vi "Go_To_Level.vi"(6 "Low Range":T2, 7 "High Range":T1, 9 "Go to Level":dbl, 10 "EncoderDevRef":T12={"DevStatus"={"status"=FALSE, "code"=0, "source"=""}, "EncoderIndex"=enum."Invalid", "CounterIndex"=enum."Invalid", "DistancePerCount"=1.0, "Decoding Type"=enum."4x"}, 11 "MotorControlDevRef":T3={"DeviceStatus"={"status"=FALSE, "code"=0, "source"=""}, "Type"=enum."PWM", "PWM"={"Controller"=enum."Controller 1", "PWM Channel"=enum."Invalid", "DeadBand"={"Name"="", "maxPositivePwm"=0, "minPositivePwm"=0, "centerPwm"=0, "maxNegativePwm"=0, "minNegativePwm"=0, "angularRange"=0}}, "CAN"={"Device Number"=0, "Control Mode"=enum."Percent VBus", "Semaphore"=refnum, "Max Vout"=12.0, "TalonSRX Control Mode"=enum."Percent VBus"}, "Invert"=FALSE, "TransformRef"=refnum, "InvTransformRef"=refnum}) -> ()   [LabVIEW 2014]
uses:
  <vilib>/Rock Robotics/SystemInterfaces/Encoder/FPGA_EncoderIdx.ctl
  <vilib>/Rock Robotics/WPI/Encoder/WPI_EncoderType.ctl
  <vilib>/Rock Robotics/SystemInterfaces/Counter/FPGA_CounterCtrSystemIndex.ctl
  <vilib>/Rock Robotics/WPI/Encoder/WPI_EncoderDevRef.ctl
  <vilib>/Rock Robotics/WPI/PWM/WPI_PWMTransform_ConPane.ctl
  <vilib>/Rock Robotics/WPI/CAN/Jaguar/SubVIs/WPI_CANJaguar_ControlMode.ctl
  <vilib>/Rock Robotics/WPI/CAN/TalonSRX/WPI_CANTalonSRX_APIControlMode.ctl
  <vilib>/Rock Robotics/SystemInterfaces/Typedef/FPGA_TypedefDigitalModule.ctl
  <vilib>/Rock Robotics/SystemInterfaces/DIO/FPGA_DIOPWMChannel.ctl
  <vilib>/Rock Robotics/WPI/PWM/WPI_PWMDeadband.ctl
  <vilib>/Rock Robotics/WPI/MotorControl/WPI_MotorControlType.ctl
  <vilib>/Rock Robotics/WPI/MotorControl/WPI_MotorControlDeviceRef.ctl
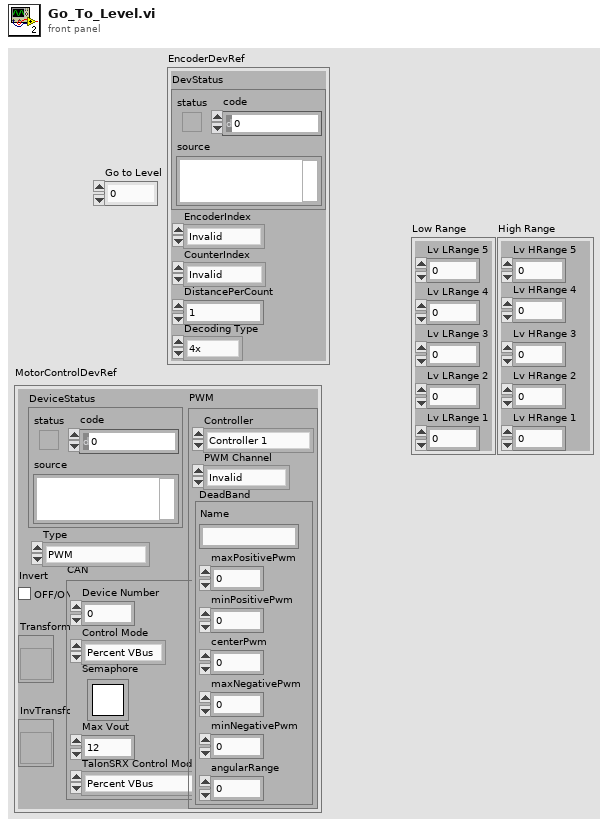
[diagram p1: front panel]
types:
  T1 = cluster{"Lv HRange 5":dbl, "Lv HRange 4":dbl, "Lv HRange 3":dbl, "Lv HRange 2":dbl, "Lv HRange 1":dbl}
  T2 = cluster{"Lv LRange 1":dbl, "Lv LRange 2":dbl, "Lv LRange 3":dbl, "Lv LRange 4":dbl, "Lv LRange 5":dbl}
  T3 = typedef "WPI_MotorControlDeviceRef.ctl" = cluster{"DeviceStatus":errorcluster, "Type":T4, "PWM":cluster{"Controller":T5, "PWM Channel":T6, "DeadBand":T7}, "CAN":cluster{"Device Number":u8, "Control Mode":T8, "Semaphore":T9, "Max Vout":dbl, "TalonSRX Control Mode":T10}, "Invert":bool, "TransformRef":T11, "InvTransformRef":T11}
  T4 = typedef "WPI_MotorControlType.ctl" = enum16{"PWM", "CAN", "CANTalonSRX"}
  T5 = typedef "FPGA_TypedefDigitalModule.ctl" = enum16{"Controller 1"}
  T6 = typedef "FPGA_DIOPWMChannel.ctl" = enum8{"PWM 0", "PWM 1", "PWM 2", "PWM 3", "PWM 4", "PWM 5", "PWM 6", "PWM 7", "PWM 8", "PWM 9", "PWM MXP 0", "PWM MXP 1", "PWM MXP 2", "PWM MXP 3", "PWM MXP 4", "PWM MXP 5", "PWM MXP 6", "PWM MXP 7", "PWM MXP 8", "PWM MXP 9", "Invalid"}
  T7 = typedef "WPI_PWMDeadband.ctl" = cluster{"Name":string, "maxPositivePwm":i32, "minPositivePwm":i32, "centerPwm":i32, "maxNegativePwm":i32, "minNegativePwm":i32, "angularRange":u16}
  T8 = typedef "WPI_CANJaguar_ControlMode.ctl" = enum8{"Percent VBus", "Current", "Speed", "Position", "Voltage"}
  T9 = typedef "Semaphore RefNum" = refnum<k1>
  T10 = typedef "WPI_CANTalonSRX_APIControlMode.ctl" = enum8{"Percent VBus", "Speed", "Position", "Slave", "Unchanged / Invalid"}
  T11 = typedef "WPI_PWMTransform_ConPane.ctl" = refnum<vi>
  T12 = typedef "WPI_EncoderDevRef.ctl" = cluster{"DevStatus":errorcluster, "EncoderIndex":T13, "CounterIndex":T14, "DistancePerCount":dbl, "Decoding Type":T15}
  T13 = typedef "FPGA_EncoderIdx.ctl" = enum8{"Enc 0", "Enc 1", "Enc 2", "Enc 3", "Enc 4", "Enc 5", "Enc 6", "Enc 7", "Invalid"}
  T14 = typedef "FPGA_CounterCtrSystemIndex.ctl" = enum8{"Ctr 0", "Ctr 1", "Ctr 2", "Ctr 3", "Ctr 4", "Ctr 5", "Ctr 6", "Ctr 7", "Invalid"}
  T15 = typedef "WPI_EncoderType.ctl" = enum16{"1x", "2x", "4x"}
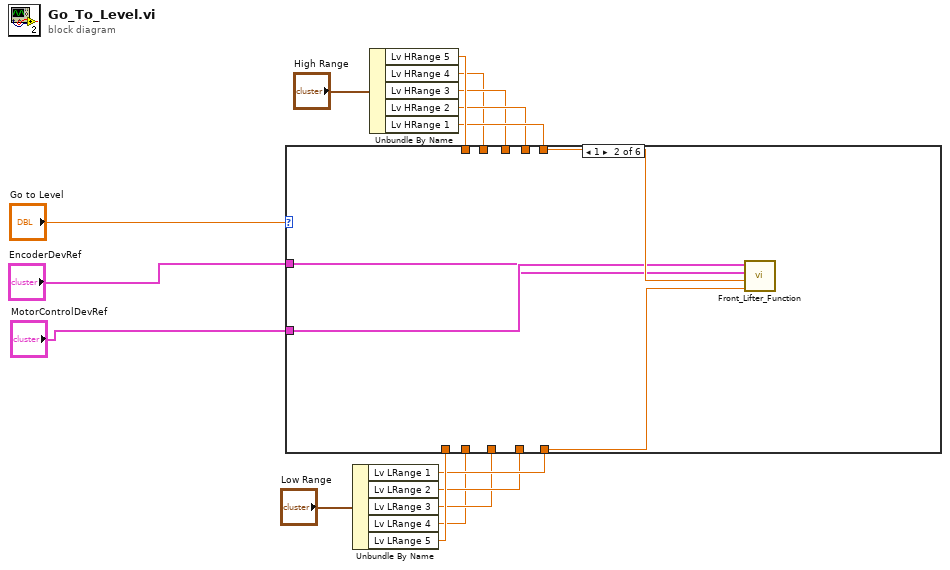
[diagram p0: block diagram]
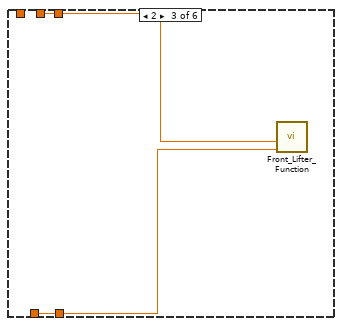
[diagram p3: hidden frame]
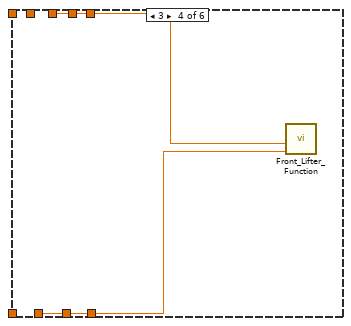
[diagram p4: hidden frame]
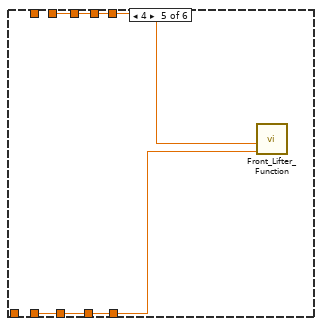
[diagram p5: hidden frame]
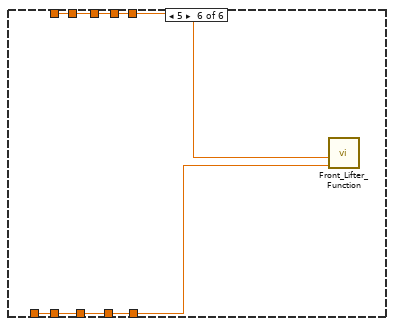
[diagram p6: hidden frame]
diagram:
  n1 = Unbundle By Name("Low Range") -> ("Lv LRange 1"=w8:dbl, "Lv LRange 2"=w6:dbl, "Lv LRange 3"=w4:dbl, "Lv LRange 4"=w1:dbl, "Lv LRange 5"=w9:dbl)
  n2 = Unbundle By Name("High Range") -> ("Lv HRange 5"=w10:dbl, "Lv HRange 4"=w2:dbl, "Lv HRange 3"=w3:dbl, "Lv HRange 2"=w5:dbl, "Lv HRange 1"=w7:dbl)
  n3 = case shown="1" "Go to Level" {
    tunnel: "EncoderDevRef" -> [_ w16 _ _ _ _]
    tunnel: "MotorControlDevRef" -> [_ w17 _ _ _ _]
    tunnel: w10 -> [_ _ _ _ _ w27]
    tunnel: w9 -> [_ _ _ _ _ w26]
    tunnel: w8 -> [_ w19 _ _ _ _]
    tunnel: w7 -> [_ w18 _ _ _ _]
    tunnel: w6 -> [_ _ w21 _ _ _]
    tunnel: w5 -> [_ _ w20 _ _ _]
    tunnel: w4 -> [_ _ _ w23 _ _]
    tunnel: w3 -> [_ _ _ w22 _ _]
    tunnel: w2 -> [_ _ _ _ w25 _]
    tunnel: w1 -> [_ _ _ _ w24 _]
    frame 0, Default {
    }
    frame 1 {
      n4 = call "Front_Lifter_Function.vi"(8:w19, 9:w18, "Go to Level?"=w16, 11:w17) -> ()  [unwired: 6 in, 2 out]
    }
    frame 2 {
      n5 = call "Front_Lifter_Function.vi"(8:w21, 9:w20) -> ()  [unwired: 8 in, 2 out]
    }
    frame 3 {
      n6 = call "Front_Lifter_Function.vi"(8:w23, 9:w22) -> ()  [unwired: 8 in, 2 out]
    }
    frame 4 {
      n7 = call "Front_Lifter_Function.vi"(8:w24, 9:w25) -> ()  [unwired: 8 in, 2 out]
    }
    frame 5 {
      n8 = call "Front_Lifter_Function.vi"(8:w26, 9:w27) -> ()  [unwired: 8 in, 2 out]
    }
  }
